vi "TSC Material Theme Tag--constant.vi"() -> (3 "Theme Path Tag":string)   [LabVIEW 2021, in "Material SubVIs.lvlib"]
doc: "CONSTANT VI - defines the user VI tag for the theme path\n\n<b>Code Developed By:</b> +\nDaniel Coons +\nTechnology Service Corporation +\nwww.tsc.com/atcs"
uses:
  Material SubVIs.lvlib
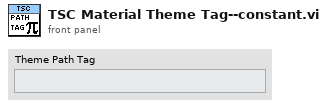
[diagram p1: front panel]
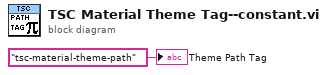
[diagram p0: block diagram]
diagram:
  "Theme Path Tag" <- "tsc-material-theme-path" ("Theme Path Tag")
